vi "make magnet graphs with correction.vi"(7 "triggered?":bool, 9 "graph type":T2(ring), 10 "rbar_parallel":dbl[](array[numeric]), 11 "mag no drive":T3[](array[typedef])) -> (0 "mag time graphs":cluster{dbl[], dbl[]}[](array[cluster]), 1 "angle":dbl, 2 "mag pos axes limits":cluster{"mag pos max":dbl, "mag pos min":dbl}, 3 "mag position graphs":T1(array[cluster]), 4 "signed area":dbl)   [LabVIEW 2017]
uses:
  typedefs/reading3.ctl
  <vilib>/Analysis/6fits.llb/Curve Fitting Criteria.ctl
  <vilib>/Analysis/baseanly.llb/Mean (DBL).vi
  <vilib>/Analysis/NI_AALBase.lvlib
  <vilib>/Analysis/NI_AALPro.lvlib
  <vilib>/Analysis/NI_AAL_Geometry.lvlib
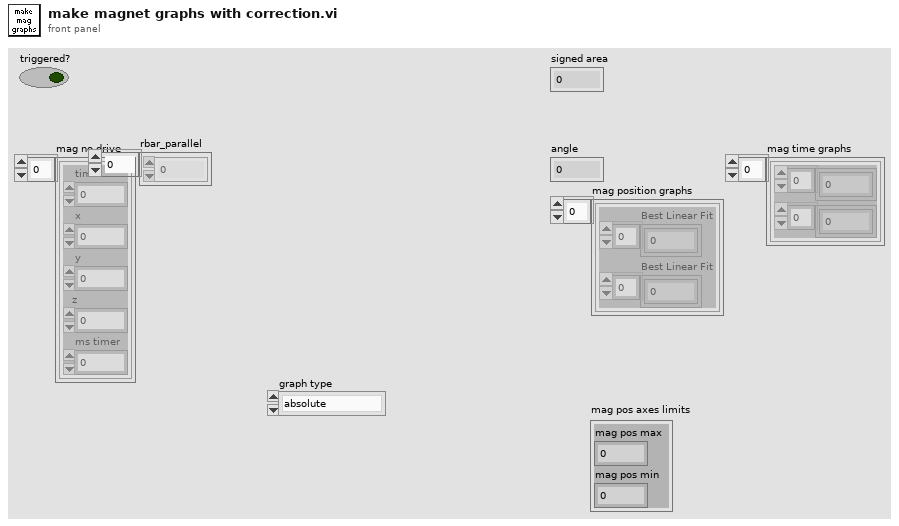
[diagram p1: front panel]
types:
  T1 = cluster{"Best Linear Fit":dbl[], "Best Linear Fit":dbl[]}[]
  T2 = enum16{"absolute", "relative", "positional", "position only"}
  T3 = typedef "reading3.ctl" = cluster{"time":dbl, "x":dbl, "y":dbl, "z":dbl, "ms timer":u32}
  T4 = typedef "NI_AALPro.lvlib/Curve Fitting Criteria.ctl" = u16
  T5 = cluster{"time":dbl, "x":dbl, "y":dbl, "z":dbl, "ms timer":dbl}
  T6 = cluster{"Best Linear Fit":dbl[], "Best Linear Fit":dbl[]}
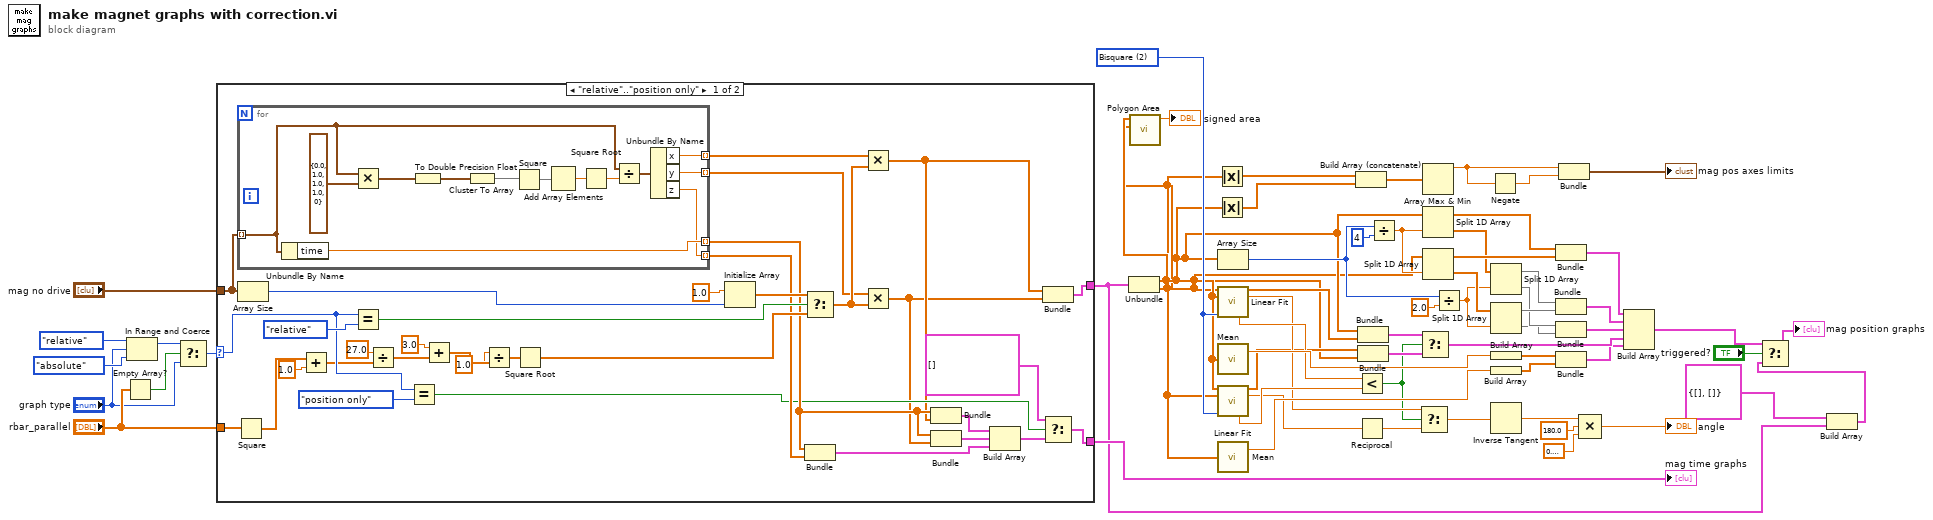
[diagram p0: block diagram]
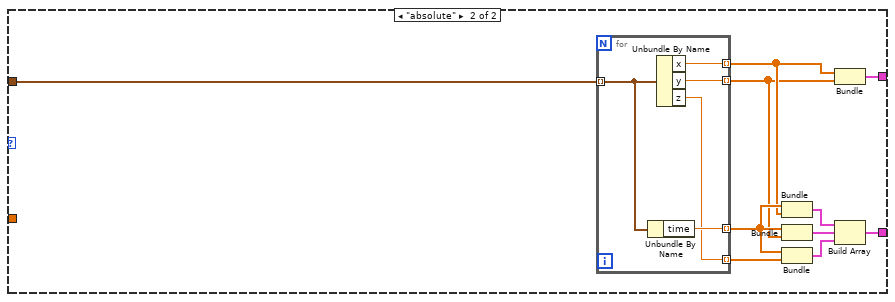
[diagram p2: hidden frame]
diagram:
  w34 = T4 2 items=["Least Square", "Least Absolute Residual", "Bisquare"] ("method")
  n1 = Empty Array?(array="rbar_parallel") -> (empty?=w13:bool)
  n2 = In Range and Coerce(upper limit=T2."relative", x="graph type", lower limit=T2."absolute") -> (coerced(x)=w12:T2)  [unwired: 1 out]
  n3 = Select(t=w12, s=w13, f="graph type") -> (s? t:f=w10:T2)
  n4 = case shown="\"relative\"..\"position only\"" w10 {
    selector: w10 -> [w72 _]
    tunnel: "mag no drive" -> [w65 w119]
    tunnel: "rbar_parallel" -> [w89 _]
    tunnel: [w74 w114] -> w7
    tunnel: [w68 w110] -> w23
    frame "relative".."position only" {
      n5 = Square(x=w89) -> (x^2=w94:dbl[])
      n6 = for {
        tunnel: w65 -> [w101] mode=indexing
        tunnel: [w98] -> w76 mode=indexing
        tunnel: [w97] -> w75 mode=indexing
        tunnel: [w104] -> w78 mode=indexing
        tunnel: [w100] -> w77 mode=indexing
        n7 = Unbundle By Name(w101) -> ("time"=w104:dbl)
        n8 = Multiply(x=w101, y=T3 {"time"=0.0, "x"=1.0, "y"=1.0, "z"=1.0, "ms timer"=0}) -> (x*y=w103:T3)
        n9 = To Double Precision Float(number=w103) -> (double precision float=w102:T5)
        n10 = Cluster To Array(cluster=w102) -> (array=w109:dbl[])
        n11 = Square(x=w109) -> (x^2=w108:dbl[])
        n12 = Add Array Elements(numeric array=w108) -> (sum=w107:dbl)
        n13 = Square Root(x=w107) -> (sqrt(x)=w106:dbl)
        n14 = Divide(x=w101, y=w106) -> (x/y=w99:T5)
        n15 = Unbundle By Name(w99) -> ("x"=w98:dbl, "y"=w97:dbl, "z"=w100:dbl)
      }
      n16 = Array Size(array=w65) -> (size(s)=w88:i32)
      n17 = Add(x=w94, y=1.0) -> (x+y=w67:dbl[])
      n18 = Equal?(x=w72, y=T2."relative") -> (x = y?=w85:bool)
      n19 = Divide(x=27.0, y=w67) -> (x/y=w93:dbl[])
      n20 = Equal?(x=w72, y=T2."position only") -> (x = y?=w70:bool)
      n21 = Add(x=3.0, y=w93) -> (x+y=w96:dbl[])
      n22 = Divide(x=1.0, y=w96) -> (x/y=w95:dbl[])
      n23 = Square Root(x=w95) -> (sqrt(x)=w83:dbl[])
      n24 = Initialize Array(1.0, w88) -> (w84:dbl[])
      n25 = Select(t=w84, s=w85, f=w83) -> (s? t:f=w82:dbl[])
      n26 = Bundle(w78, w77) -> (w79:cluster{dbl[], dbl[]})  [unwired: 1 in]
      n27 = Multiply(x=w76, y=w82) -> (x*y=w64:dbl[])
      n28 = Multiply(x=w75, y=w82) -> (x*y=w63:dbl[])
      n29 = Bundle(w78, w64) -> (w81:cluster{dbl[], dbl[]})  [unwired: 1 in]
      n30 = Bundle(w78, w63) -> (w80:cluster{dbl[], dbl[]})  [unwired: 1 in]
      n31 = Build Array(w81, w80, w79) -> (w73:cluster{dbl[], dbl[]}[])
      n32 = Bundle(w64, w63) -> (w74:cluster{dbl[], dbl[]})  [unwired: 1 in]
      n33 = Select(t=cluster{dbl[], dbl[]}[] [], s=w70, f=w73) -> (s? t:f=w68:cluster{dbl[], dbl[]}[])
    }
    frame "absolute" {
      n34 = for {
        tunnel: w119 -> [w120] mode=indexing
        tunnel: [w124] -> w116 mode=indexing
        tunnel: [w123] -> w115 mode=indexing
        tunnel: [w122] -> w118 mode=indexing
        tunnel: [w121] -> w117 mode=indexing
        n35 = Unbundle By Name(w120) -> ("time"=w122:dbl)
        n36 = Unbundle By Name(w120) -> ("x"=w124:dbl, "y"=w123:dbl, "z"=w121:dbl)
      }
      n37 = Bundle(w118, w116) -> (w113:cluster{dbl[], dbl[]})  [unwired: 1 in]
      n38 = Bundle(w118, w115) -> (w112:cluster{dbl[], dbl[]})  [unwired: 1 in]
      n39 = Bundle(w118, w117) -> (w111:cluster{dbl[], dbl[]})  [unwired: 1 in]
      n40 = Bundle(w116, w115) -> (w114:cluster{dbl[], dbl[]})  [unwired: 1 in]
      n41 = Build Array(w113, w112, w111) -> (w110:cluster{dbl[], dbl[]}[])
    }
  }
  "mag time graphs" <- w23
  n42 = Unbundle(w7) -> (w3:dbl[], w2:dbl[])
  n43 = call <vilib>:"Polygon Area.vi"("Y"=w2, "X"=w3) -> ("signed area"=→"signed area":dbl)  [unwired: 8 in, 1 out]
  n44 = Absolute Value(x=w2) -> (abs(x)=w21:dbl[])
  n45 = Absolute Value(x=w3) -> (abs(x)=w22:dbl[])
  n46 = Array Size(array=w3) -> (size(s)=w50:i32)
  n47 = call <vilib>:"Linear Fit.vi"("Y"=w2, "X"=w3, "method"=w34) -> ("Best Linear Fit"=w26:dbl[], "slope"=w31:dbl, "residue"=w32:dbl)  [unwired: 8 in, 2 out]
  n48 = call-poly <vilib>:"Mean.vi"("X"=w3) -> ("mean"=w42:dbl)  [unwired: 1 out]
  n49 = call <vilib>:"Linear Fit.vi"("Y"=w3, "X"=w2, "method"=w34) -> ("Best Linear Fit"=w25:dbl[], "slope"=w29:dbl, "residue"=w33:dbl)  [unwired: 8 in, 2 out]
  n50 = call-poly <vilib>:"Mean.vi"("X"=w2) -> ("mean"=w41:dbl)  [unwired: 1 out]
  n51 = Build Array (concatenate)(w21, w22) -> (w20:dbl[])
  n52 = Less?(x=w32, y=w33) -> (x < y?=w27:bool)
  n53 = Reciprocal(x=w29) -> (1/x=w28:dbl)
  n54 = Bundle(w3, "Best Linear Fit"=w26) -> (w61:cluster{dbl[], "Best Linear Fit":dbl[]})  [unwired: 1 in]
  n55 = Bundle("Best Linear Fit"=w25, w2) -> (w59:cluster{"Best Linear Fit":dbl[], dbl[]})  [unwired: 1 in]
  n56 = Divide(x=w50, y=4) -> (x/y=w57:dbl)
  n57 = Select(t=w31, s=w27, f=w28) -> (s? t:f=w30:dbl)
  n58 = Select(t=w61, s=w27, f=w59) -> (s? t:f=w60:T6)
  n59 = Array Max & Min(array=w20) -> (max value=w18:dbl)  [unwired: 3 out]
  n60 = Split 1D Array(array=w3, index=w57) -> (first subarray=w56:dbl[], second subarray=w53:dbl[])
  n61 = Split 1D Array(array=w2, index=w57) -> (first subarray=w55:dbl[], second subarray=w52:dbl[])
  n62 = Divide(x=w50, y=2.0) -> (x/y=w49:dbl)
  n63 = Negate(x=w18) -> (-x=w19:dbl)
  n64 = Split 1D Array(array=w53, index=w49) -> (first subarray=w48:dbl[], second subarray=w46:dbl[])
  n65 = Split 1D Array(array=w52, index=w49) -> (first subarray=w47:dbl[], second subarray=w45:dbl[])
  n66 = Build Array(w42) -> (w40:dbl[])
  n67 = Build Array(w41) -> (w39:dbl[])
  n68 = Inverse Tangent(1:w30) -> (0:w37:dbl)
  n69 = Bundle(w56, w55) -> (w54:cluster{dbl[], dbl[]})  [unwired: 1 in]
  n70 = Bundle(w48, w47) -> (w44:cluster{dbl[], dbl[]})  [unwired: 1 in]
  n71 = Bundle(w46, w45) -> (w43:cluster{dbl[], dbl[]})  [unwired: 1 in]
  n72 = Bundle(w40, w39) -> (w38:cluster{dbl[], dbl[]})  [unwired: 1 in]
  n73 = Bundle(w18, w19) -> (→"mag pos axes limits":cluster{dbl, dbl})  [unwired: 1 in]
  n74 = Compound Arithmetic op=MULTIPLY(w37, 180.0 ("y"), 0.3183098861837907) -> (→"angle":dbl)
  n75 = Build Array(w54, w44, w43, w60, w38) -> (w9:T1)
  n76 = Build Array(cluster{dbl[], dbl[]} {[], []} ("element"), w7) -> (w5:cluster{dbl[], dbl[]}[])
  n77 = Select(t=w9, s="triggered?", f=w5) -> (s? t:f=→"mag position graphs":T1)
